vi "Load DAC Configuration.vi"(8 "error in":errorcluster, 10 "Config File refnum in":T1, 11 "DAC Vacum Valve in":refnum<class "DAC Vacum Valve.lvclass"> caption="DAC Heater dU in") -> (0 "error out":errorcluster, 2 "Config File refnum out":T1, 3 "DAC Vacum Valve out":refnum<class "DAC Vacum Valve.lvclass">)   [LabVIEW 2019, in "DAC.lvlib" / "DAC Vacum Valve.lvclass"]
uses:
  DAC Vacum Valve.lvclass
  C:/Users/krio/Documents/LV_Projects/test-stand/App/DAC/DAC.lvclass
  <vilib>/Utility/config.llb/Config Data RefNum.ctl
  DAC.lvclass/DAC.ctl
  DAC Vacum Valve.lvclass/DAC Vacum Valve.ctl
  <vilib>/Utility/config.llb/Read Key (String).vi
  DAC.lvclass
  <vilib>/Utility/config.llb/NI_LVConfig.lvlib
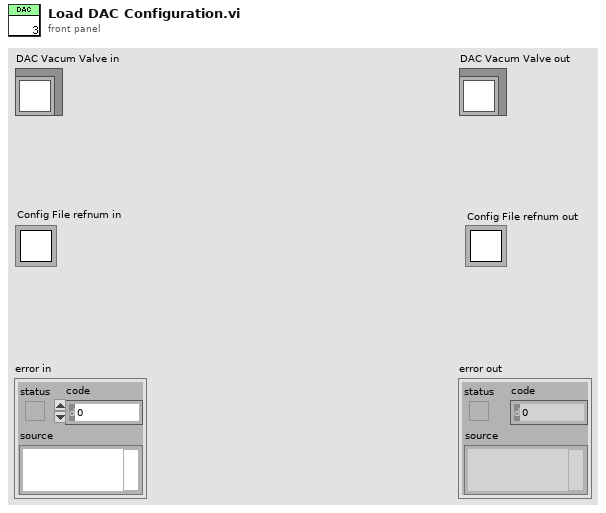
[diagram p1: front panel]
types:
  T1 = typedef "NI_LVConfig.lvlib/Config Data RefNum.ctl" = refnum<k1>
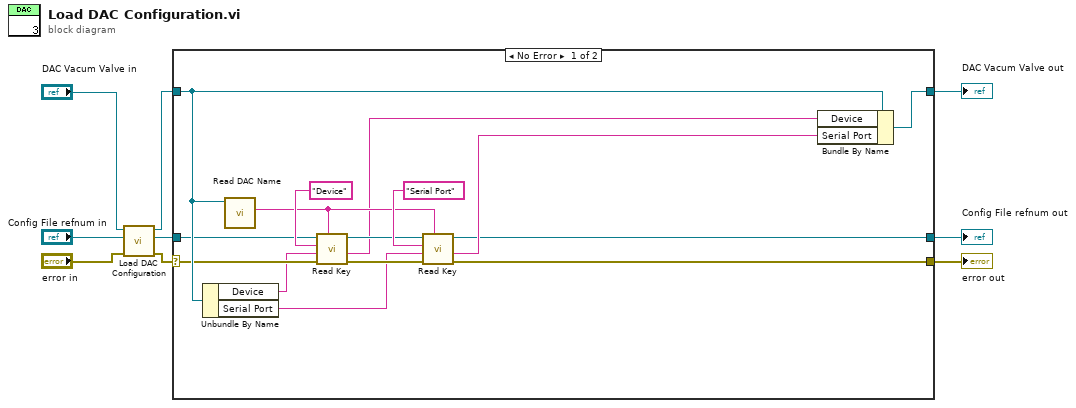
[diagram p0: block diagram]
diagram:
  n1 = call-parent "Load DAC Configuration.vi"("error in"="error in", "Config File refnum in"="Config File refnum in", "DAC in"="DAC Vacum Valve in") -> ("error out"=w4:errorcluster, "Config File refnum out"=w5:T1, "DAC out"=w6:refnum<class "DAC Vacum Valve.lvclass">)  [unwired: 6 in]
  n2 = case shown="No Error" w4 {
    selector: w4 -> [w18 w27]
    tunnel: [w10 w27] -> w1
    tunnel: [w24 w26] -> w3
    tunnel: w6 -> [w23 w26]
    tunnel: w5 -> [w19 w25]
    tunnel: [w11 w25] -> w2
    frame No Error {
      n3 = Unbundle By Name(w23) -> ("Device"=w16:string, "Serial Port"=w14:string)
      n4 = call "Read DAC Name.vi"("DAC in"=w23) -> ("DAC Name"=w15:string)  [unwired: 8 in, 2 out]
      n5 = call-poly <vilib>:"Read Key.vi"("section"=w15, "error in (no error)"=w18, "default value"=w16, "key"="Device", "refnum"=w19) -> ("error out"=w17:errorcluster, "value"=w13:string, "refnum out"=w20:T1)  [unwired: 3 in, 1 out]
      n6 = call-poly <vilib>:"Read Key.vi"("section"=w15, "error in (no error)"=w17, "default value"=w14, "key"="Serial Port", "refnum"=w20) -> ("error out"=w10:errorcluster, "value"=w12:string, "refnum out"=w11:T1)  [unwired: 3 in, 1 out]
      n7 = Bundle By Name(cluster=w23, "Device"=w13, "Serial Port"=w12) -> (w24:refnum<class "DAC Vacum Valve.lvclass">)
    }
    frame Error {
    }
  }
  "error out" <- w1
  "DAC Vacum Valve out" <- w3
  "Config File refnum out" <- w2
